vi "Push_Wrapping.vi"   [LabVIEW 2024, in "POTCircularBuffer.Tests.Units.lvlib"]
uses:
  POTCircularBuffer.Tests.Units.lvlib
  Type.ctl
  POTTypedCircularBuffer.lvclass/POTTypedCircularBuffer.ctl
  Wrap.vi
  ReadCount.vi
  Reorder.vi
  Flush.vi
  <vilib>/addons/_JKI Toolkits/Caraya/classes/Assert/Assert Equal Value_Variant.vi
  <vilib>/addons/_JKI Toolkits/Caraya/classes/Test/Test.lvclass
  <vilib>/addons/_JKI Toolkits/Caraya/classes/Assert/Assert.lvclass
  POTTypedCircularBuffer.lvclass
types:
  T1 = typedef "POTTypedCircularBuffer.lvclass/Type.ctl" = i32
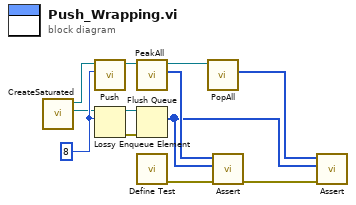
[diagram p0: block diagram]
diagram:
  w8 = T1 8 ("Element")
  n1 = call "CreateSaturated.vi"() -> ("Golden"=w4:refnum<queue>, "POTTypedCircularBuffer out"=w2:refnum<class "POTTypedCircularBuffer.lvclass">)  [unwired: 10 in]
  n2 = call "Push.vi"("Element"=w8, "POTTypedCircularBuffer in"=w2) -> ("POTTypedCircularBuffer out"=w1:refnum<class "POTTypedCircularBuffer.lvclass">)  [unwired: 9 in]
  n3 = Lossy Enqueue Element(queue=w4, element=w8) -> (queue out=w6:refnum<queue>, error out=w7:errorcluster)  [unwired: 1 in, 2 out]
  n4 = call "PeakAll.vi"("POTTypedCircularBuffer in"=w1) -> ("Copied Buffer"=w11:T1[], "POTTypedCircularBuffer out"=w10:refnum<class "POTTypedCircularBuffer.lvclass">)  [unwired: 9 in]
  n5 = Flush Queue(queue=w6, error in (no error)=w7) -> (remaining elements=w3:T1[])  [unwired: 2 out]
  n6 = call <vilib>:"Define Test.vi"() -> ("error out"=w12:errorcluster)  [unwired: 10 in, 1 out]
  n7 = call "PopAll.vi"("POTTypedCircularBuffer in"=w10) -> ("Flushed Buffer"=w5:T1[])  [unwired: 9 in, 1 out]
  n8 = call-poly <vilib>:"Assert.vi"("error in (no error)"=w12, "Y"=w3, "X"=w11) -> ("error out"=w9:errorcluster)  [unwired: 7 in, 1 out]
  n9 = call-poly <vilib>:"Assert.vi"("error in (no error)"=w9, "Y"=w3, "X"=w5) -> ()  [unwired: 7 in, 2 out]
